vi "Teleop.vi"(9 "comm in":refnum<notifier>, 10 "Match Info":T1={"Autonomous Elapsed Seconds"=0.0, "TeleOp Elapsed Seconds"=0.0, "Disabled Elapsed Seconds"=0.0, "Visited Autonomous"=FALSE, "Visited TeleOp"=FALSE, "Visited Disabled"=FALSE, "Autonomous Settings"={"Autonomous Style"=enum."Independent", "VI Refnum"=refnum}}, 11 "Call Context":T2) -> ()   [LabVIEW 2015]
doc: "This VI is called for each TeleOp packet received from the DS where the robot is not disabled. It is often used to read from the joysticks and update I/O or to update setpoints for timed control loops. It should complete and return within 20 milliseconds or it may miss DS packets."
uses:
  <vilib>/Rock Robotics/WPI/DriverStation/WPI_DriverStationDerivedRobotMode.ctl
  <vilib>/Rock Robotics/WPI/DriverStation/WPI_DriverStationMatch Info.ctl
  Downloads/basic commandNcontrol/basic commandNcontrol/commands.ctl
  <vilib>/Rock Robotics/WPI/Utilities/WPI_GetSetVariantRefNum.vi
  <vilib>/Rock Robotics/Network Tables/NT Write Boolean Array.vi
  <vilib>/Rock Robotics/Network Tables/NT Write Numeric Array.vi
  <vilib>/Rock Robotics/Network Tables/NT Read Boolean.vi
  <vilib>/Rock Robotics/Network Tables/NT Read Number.vi
panel:
  out "Buttons":bool[](array[boolean])
  out "Sample Slider 0":dbl(slide) scale=0.0..5.0
  out "Sample Boolean 1":bool
  out "Sample Boolean 0":bool
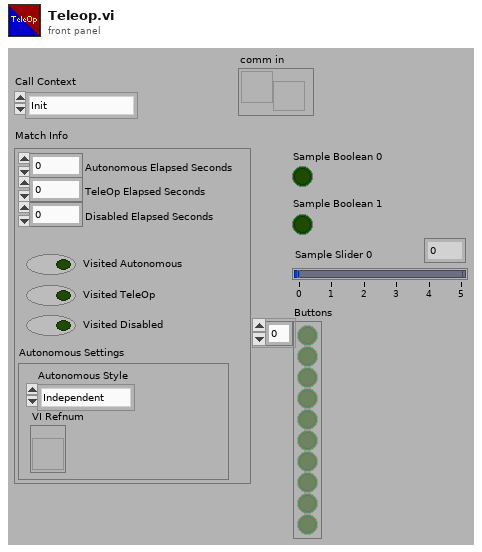
[diagram p1: front panel]
types:
  T1 = typedef "WPI_DriverStationMatch Info.ctl" = cluster{"Autonomous Elapsed Seconds":dbl, "TeleOp Elapsed Seconds":dbl, "Disabled Elapsed Seconds":dbl, "Visited Autonomous":bool, "Visited TeleOp":bool, "Visited Disabled":bool, "Autonomous Settings":cluster{"Autonomous Style":enum16{"Iterative", "Independent"}, "VI Refnum":refnum<vi>}}
  T2 = typedef "WPI_DriverStationDerivedRobotMode.ctl" = enum16{"Init", "Execute", "Stop"}
  T3 = typedef "WPI_RobotDriveDevRef.ctl" = cluster{"DevStatus":errorcluster, "Motors[]":T4[], "Square Inputs":bool, "Max Output":dbl}
  T4 = typedef "WPI_MotorControlDeviceRef.ctl" = cluster{"DeviceStatus":errorcluster, "Type":T5, "PWM":cluster{"PWM Channel":T6, "DeadBand":T7}, "CAN":cluster{"Device Number":u8, "Control Mode":T8, "Semaphore":T9, "Max Vout":dbl, "TalonSRX Control Mode":T10}, "Invert":bool}
  T5 = typedef "WPI_MotorControlType.ctl" = enum16{"PWM", "CAN", "CANTalonSRX"}
  T6 = typedef "FPGA_DIOPWMChannel.ctl" = enum8{"PWM 0", "PWM 1", "PWM 2", "PWM 3", "PWM 4", "PWM 5", "PWM 6", "PWM 7", "PWM 8", "PWM 9", "PWM MXP 0", "PWM MXP 1", "PWM MXP 2", "PWM MXP 3", "PWM MXP 4", "PWM MXP 5", "PWM MXP 6", "PWM MXP 7", "PWM MXP 8", "PWM MXP 9", "Invalid"}
  T7 = typedef "WPI_PWMDeadband.ctl" = cluster{"Name":string, "maxPositivePwm":i32, "minPositivePwm":i32, "centerPwm":i32, "maxNegativePwm":i32, "minNegativePwm":i32, "angularRange":u16}
  T8 = typedef "WPI_CANJaguar_ControlMode.ctl" = enum8{"Percent VBus", "Current", "Speed", "Position", "Voltage"}
  T9 = typedef "Semaphore RefNum" = refnum<k1>
  T10 = typedef "WPI_CANTalonSRX_APIControlMode.ctl" = enum8{"Percent VBus", "Speed", "Position", "Slave", "Unchanged / Invalid", "Voltage Compensation", "Current", "Motion Profile"}
  T11 = typedef "WPI_JoystickDevRef.ctl" = cluster{"Device":T12}
  T12 = typedef "WPI_JoystickDeviceEnum.ctl" = enum16{"USB 0", "USB 1", "USB 2", "USB 3", "USB 4", "USB 5"}
  T13 = typedef "commands.ctl" = cluster{"command":enum16{"StandBy", "printHello", "printFRC", "printBalls", "exit"}, "data":variant}
  T14 = typedef "WPI_DigitalInputDevRef.ctl" = cluster{"DevStatus":errorcluster, "DIO Channel":T15}
  T15 = typedef "FPGA_DIOChannel.ctl" = enum8{"DIO 0", "DIO 1", "DIO 2", "DIO 3", "DIO 4", "DIO 5", "DIO 6", "DIO 7", "DIO 8", "DIO 9", "DIO MXP 0", "DIO MXP 1", "DIO MXP 2", "DIO MXP 3", "DIO MXP 4", "DIO MXP 5", "DIO MXP 6", "DIO MXP 7", "DIO MXP 8", "DIO MXP 9", "DIO MXP 10", "DIO MXP 11", "DIO MXP 12", "DIO MXP 13", "DIO MXP 14", "DIO MXP 15", "Invalid"}
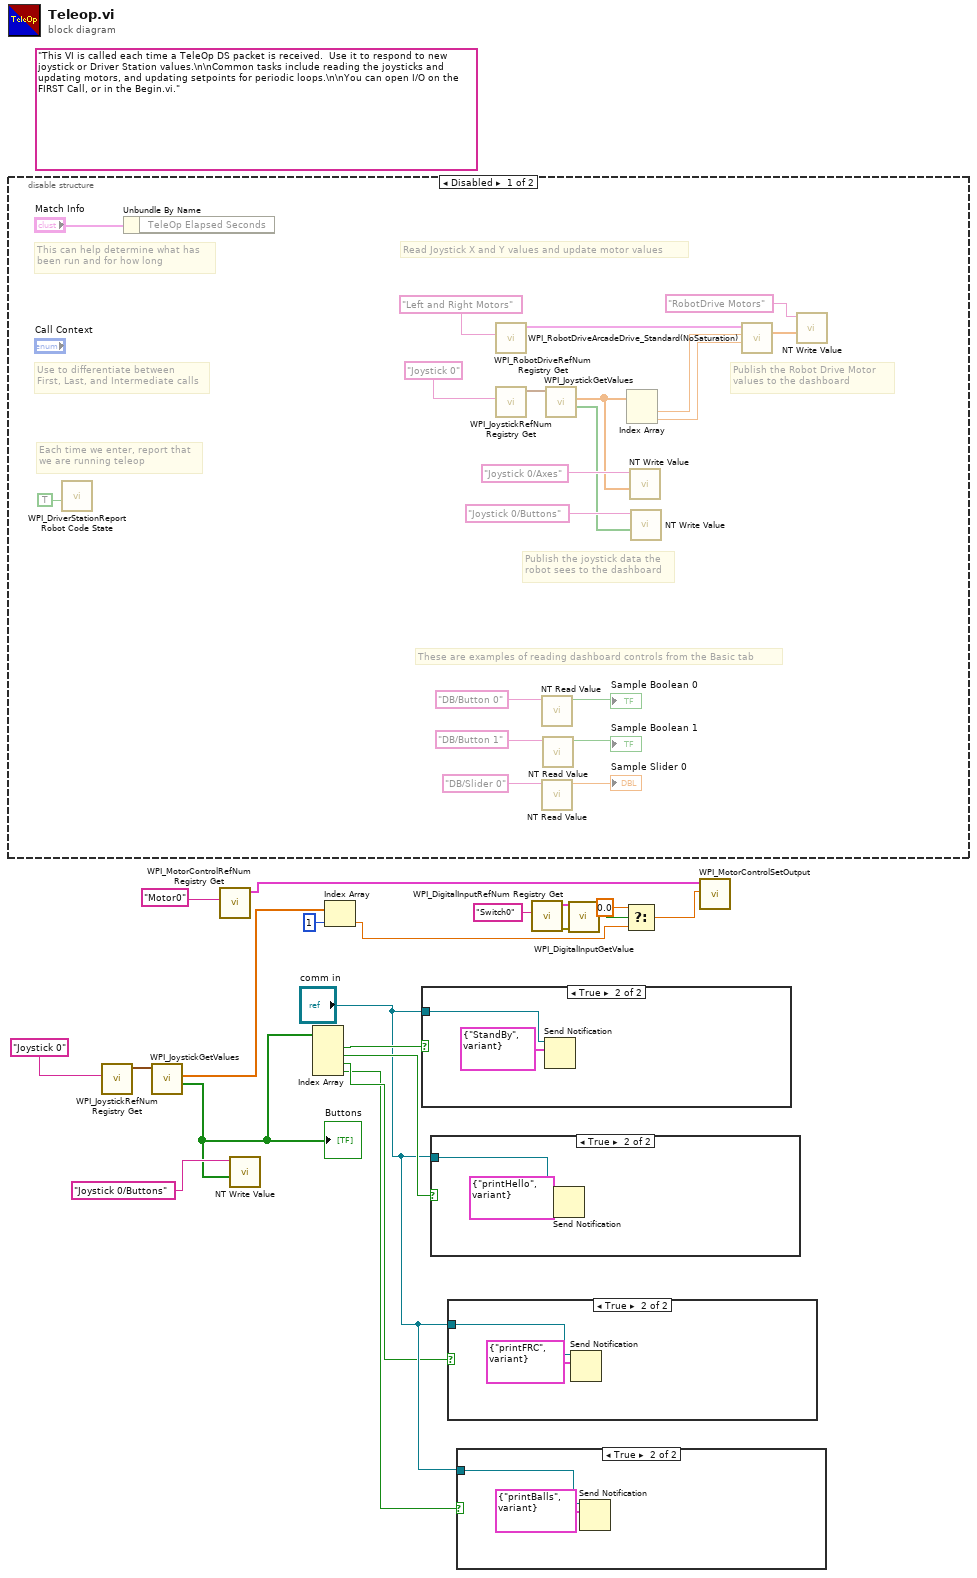
[diagram p0: block diagram]
diagram:
  (unwired) "This VI is called each time a TeleOp DS packet is received.  Use it to respond to new joystick or Driver Station values.\n\nCommon tasks include reading the joysticks and updating motors, and updating setpoints for periodic loops.\n\nYou can open I/O on the FIRST Call, or in the Begin.vi."
  n1 = disable-structure shown="Disabled" {
    frame Disabled {
      # "These are examples of reading dashboard controls from the Basic tab"
      # "Publish the Robot Drive Motor\nvalues to the dashboard"
      # "Publish the joystick data the\nrobot sees to the dashboard"
      # "Each time we enter, report that\nwe are running teleop"
      # "Use to differentiate between\nFirst, Last, and Intermediate calls"
      # "This can help determine what has\nbeen run and for how long"
      # "Read Joystick X and Y values and update motor values"
      n2 = call <vilib>:"WPI_DriverStationReport Robot Code State.vi"("TeleOp"=TRUE ("Autonomous")) -> ()  [unwired: 10 in, 1 out]
      n3 = Unbundle By Name("Match Info") -> ()  [unwired: 1 out]
      n4 = call <vilib>:"WPI_RobotDriveRefNum Registry Get.vi"("refnum name"="Left and Right Motors") -> ("RobotDriveDevRef"=w38:T3)  [unwired: 1 in, 9 out]
      n5 = call <vilib>:"WPI_JoystickRefNum Registry Get.vi"("refnum name"="Joystick 0") -> ("JoystickDevRef"=w35:T11)  [unwired: 1 in, 9 out]
      n6 = call-poly <vilib>:"NT Read Value.vi"("Name"="DB/Button 0" ("refnum name")) -> ("Boolean"=→"Sample Boolean 0":bool)  [unwired: 9 in, 1 out]
      n7 = call-poly <vilib>:"NT Read Value.vi"("Name"="DB/Slider 0" ("refnum name")) -> ("Numeric"=→"Sample Slider 0":dbl)  [unwired: 9 in, 1 out]
      n8 = call-poly <vilib>:"NT Read Value.vi"("Name"="DB/Button 1" ("refnum name")) -> ("Boolean"=→"Sample Boolean 1":bool)  [unwired: 9 in, 1 out]
      n9 = call <vilib>:"WPI_JoystickGetValues.vi"("JoystickDevRef"=w35) -> ("Buttons"=w29:bool[], "Axes"=w30:dbl[])  [unwired: 6 in, 3 out]
      n10 = Index Array(array=w30) -> (element #1=w37:dbl, element #2=w33:dbl)  [unwired: 2 in]
      n11 = call-poly <vilib>:"NT Write Value.vi"("Numeric Array"=w30, "Name"="Joystick 0/Axes") -> ()  [unwired: 9 in, 1 out]
      n12 = call-poly <vilib>:"NT Write Value.vi"("Boolean Array"=w29, "Name"="Joystick 0/Buttons") -> ()  [unwired: 9 in, 1 out]
      n13 = call <vilib>:"WPI_RobotDriveArcadeDrive_Standard(NoSaturation).vi"("Y axis value"=w33, "X axis value"=w37, "RobotDriveDevRef"=w38) -> ("Motor Values"=w22:dbl[])  [unwired: 1 in, 7 out]
      n14 = call-poly <vilib>:"NT Write Value.vi"("Numeric Array"=w22, "Name"="RobotDrive Motors") -> ()  [unwired: 9 in, 1 out]
    }
    frame Enabled {
    }
  }
  n15 = call <vilib>:"WPI_JoystickRefNum Registry Get.vi"("refnum name"="Joystick 0") -> ("JoystickDevRef"=w19:T11)  [unwired: 1 in, 9 out]
  n16 = call <vilib>:"WPI_JoystickGetValues.vi"("JoystickDevRef"=w19) -> ("Buttons"=w17:bool[], "Axes"=w8:dbl[])  [unwired: 6 in, 3 out]
  "Buttons" <- w17
  n17 = call <vilib>:"WPI_MotorControlRefNum Registry Get.vi"("refnum name"="Motor0") -> ("MotorControlDevRef"=w10:T4)  [unwired: 9 in, 1 out]
  n18 = call-poly <vilib>:"NT Write Value.vi"("Boolean Array"=w17, "Name"="Joystick 0/Buttons") -> ()  [unwired: 9 in, 1 out]
  n19 = Index Array(array=w17) -> (element #1=w16:bool, element #2=w15:bool, element #3=w13:bool, element #4=w12:bool)  [unwired: 4 in]
  n20 = Index Array(array=w8, index=1) -> (element=w2:dbl)
  n21 = case shown="True" w16 {
    tunnel: "comm in" -> [_ w42]
    frame False {
    }
    frame True {
      n22 = Send Notification(notification=T13 {"command"=enum."StandBy", "data"=variant}, notifier=w42) -> ()  [unwired: 1 in, 2 out]
    }
  }
  n23 = case shown="True" w15 {
    tunnel: "comm in" -> [_ w44]
    frame False {
    }
    frame True {
      n24 = Send Notification(notification=T13 {"command"=enum."printHello", "data"=variant}, notifier=w44) -> ()  [unwired: 1 in, 2 out]
    }
  }
  n25 = case shown="True" w13 {
    tunnel: "comm in" -> [_ w46]
    frame False {
    }
    frame True {
      n26 = Send Notification(notification=T13 {"command"=enum."printFRC", "data"=variant}, notifier=w46) -> ()  [unwired: 1 in, 2 out]
    }
  }
  n27 = case shown="True" w12 {
    tunnel: "comm in" -> [_ w48]
    frame False {
    }
    frame True {
      n28 = Send Notification(notification=T13 {"command"=enum."printBalls", "data"=variant}, notifier=w48) -> ()  [unwired: 1 in, 2 out]
    }
  }
  n29 = call <vilib>:"WPI_DigitalInputRefNum Registry Get.vi"("refnum name"="Switch0") -> ("error out"=w6:errorcluster, "DigitalInputDevRef"=w5:T14)  [unwired: 9 in]
  n30 = call <vilib>:"WPI_DigitalInputGetValue.vi"("error in (no error)"=w6, "DigitalInputDevRef"=w5) -> ("Value"=w4:bool)  [unwired: 7 in, 2 out]
  n31 = Select(t=0.0, s=w4, f=w2) -> (s? t:f=w1:dbl)
  n32 = call <vilib>:"WPI_MotorControlSetOutput.vi"("Output"=w1, "MotorControlDevRef"=w10) -> ()  [unwired: 7 in, 3 out]
